vi "VisualizeSiemensDigitalEnergyMeter.vi"() -> ()   [LabVIEW 2018, in "Visualization.lvlib" / "VisualizeSensor.lvclass"]
doc: "This VI listens for any measurement data associated with the provided PluginName and displays it to the user for analysis. The display is only suitable for data coming from the Siemens Plugin."
uses:
  VisualizeSensor.lvclass
  Sensor/SensorShared/clSensorData.ctl
  <extravilib>/ChannelInstances/Tag-bool/Write With Abort.vi
  <extravilib>/ChannelInstances/Tag-bool/Read With Abort.vi
  <extravilib>/ChannelInstances/Tag-bool/Instantiate.vi
  <extravilib>/ChannelInstances/Tag-bool/EndpointRead.vi
  <vilib>/Utility/error.llb/Error Cluster From Error Code.vi
  <extravilib>/ChannelInstances/Tag-bool/Endpoint.vi
  <vilib>/ErrorRing/Error Ring.xnode
  <userlib>/NIST/NISTErrorLib/NISTErrorLib.lvlib
  VisualizeBase/VisualizeBase_class/VisualizeBase.lvclass
  Sensor/SensorShared/SensorShared.lvlib
  Sensor/SensorModule/SensorModule.lvlib
  <extravilib>/ChannelInstances/Tag-bool.lvlib
  TestClass/Test.lvclass
panel:
  in  "ModuleID":i32
  in  "Log Data":bool=TRUE
  in  "btnStop":bool
  in  "btnReset":bool
  in  "btnClearTest":bool
  out "Siemens":waveform(dbl)[](graph)=[{"t0"=timestamp(3657200531.6397257 s since 1904-01-01), "dt"=1.0, "Y"=[46.19]}, {"t0"=timestamp(3657200531.6397257 s since 1904-01-01), "dt"=1.0, "Y"=[2.0]}, {"t0"=timestamp(3657200531.6397257 s since 1904-01-01), "dt"=1.0, "Y"=[60.0]}]
  out "ErrorArray":errorcluster[](array[cluster])
  out "Incorrect DataType?":bool
  out "String Results":string="Sensor.RoomAlert1"
  in  "PluginName":string="Sensor.RoomAlert1"
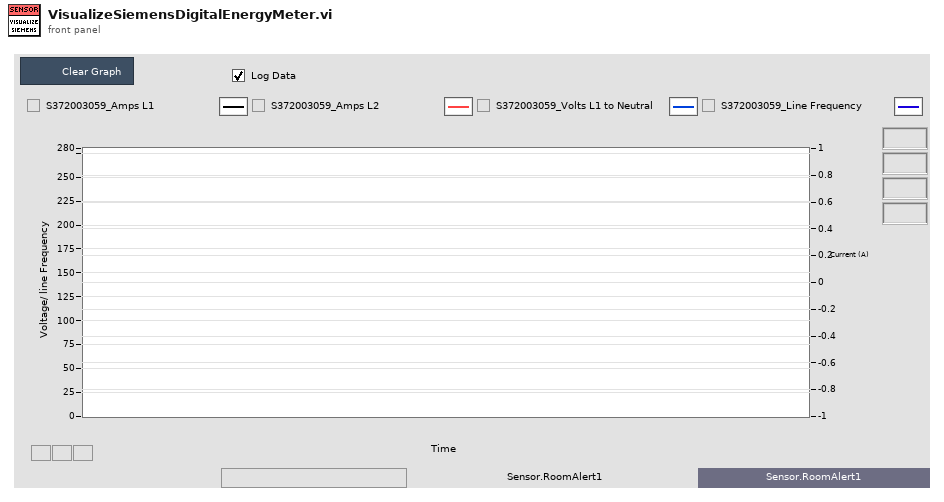
[diagram p1: front panel]
types:
  T1 = enum16{"open", "open or create", "create or replace", "create", "open (read-only)"}
  T2 = typedef "Visualization.lvlib/VisualizeBase.lvclass/clRequestEvents.ctl" = cluster{"StopRequest":refnum<user-event>, "ResetRequest":refnum<user-event>, "FP Pop In or Out":refnum<user-event>}
  T3 = typedef "SensorShared.lvlib/clBroadcastEvents.ctl" = cluster{"DidInit":refnum<user-event>, "StatusUpdate":refnum<user-event>, "ErrorReport":refnum<user-event>, "DidStop":refnum<user-event>, "PathToINI":refnum<user-event>, "SensorReport":refnum<user-event>, "SensorConfig":refnum<user-event>}
  T4 = typedef "SensorShared.lvlib/clSensorData.ctl" = cluster{"SensorType":string, "SensorData":variant}
  T5 = typedef "Tag-bool.lvlib/))Channel.ctl" = refnum<queue>
  T6 = typedef "sizeaction.ctl" = enum32{"Minimized", "Maximized", "Resized"}
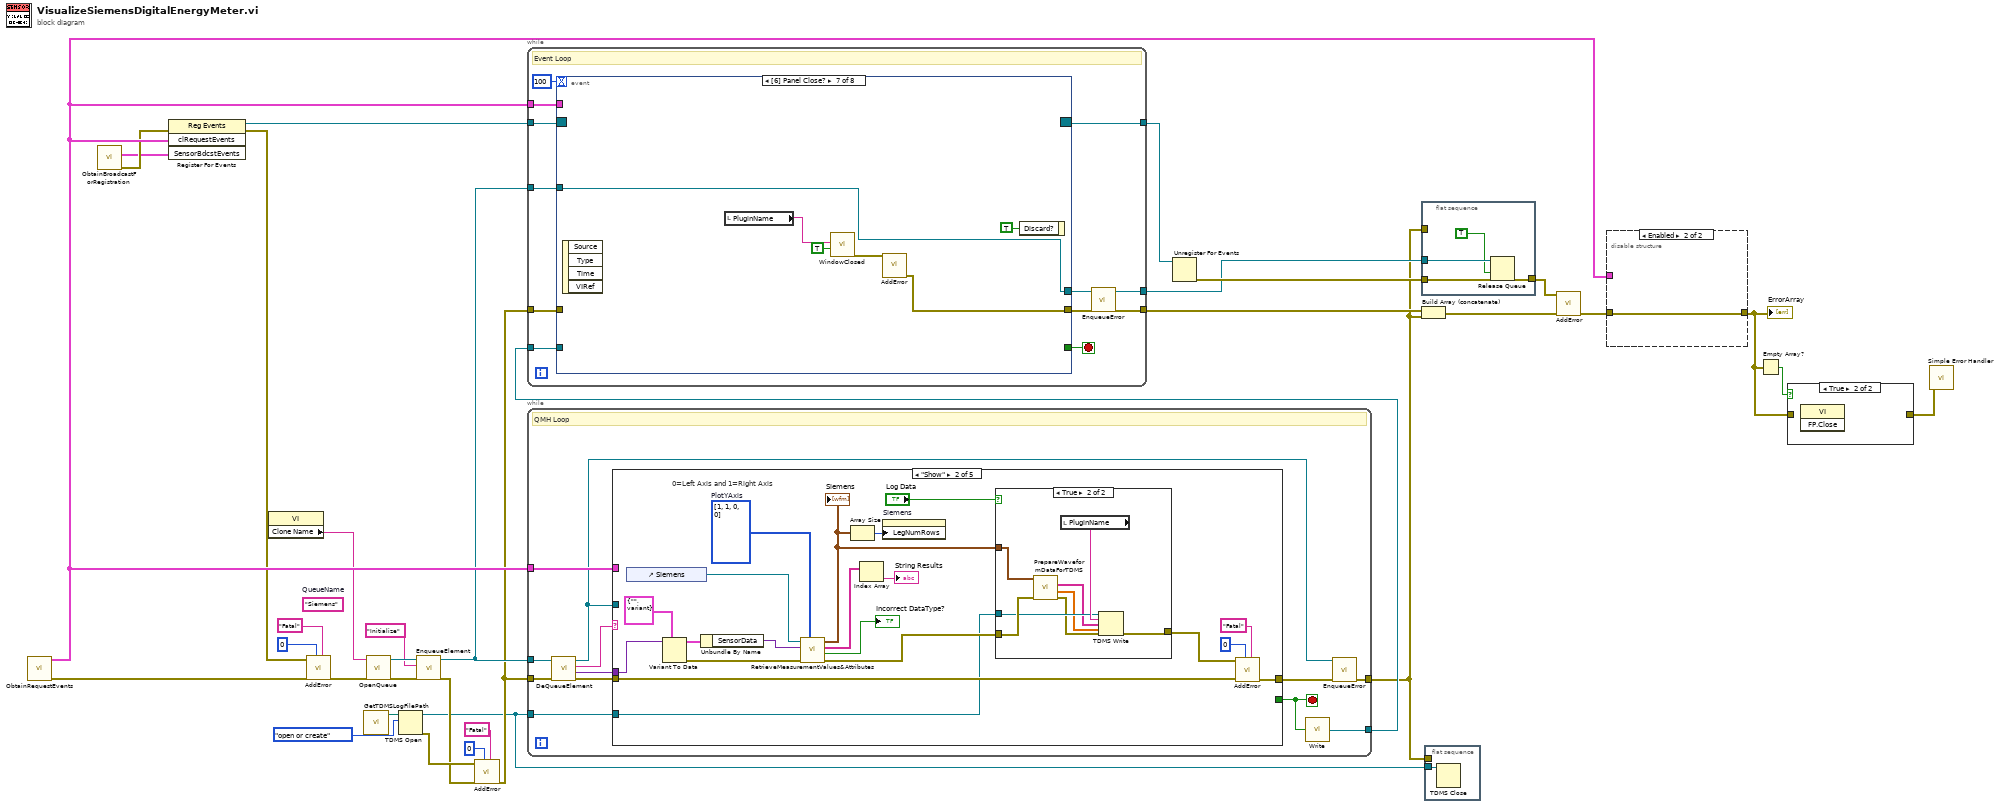
[diagram p0: block diagram]
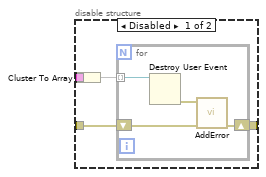
[diagram p2: hidden frame]
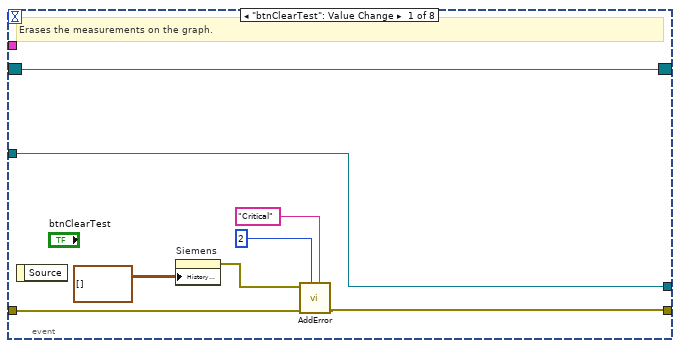
[diagram p3: hidden frame]
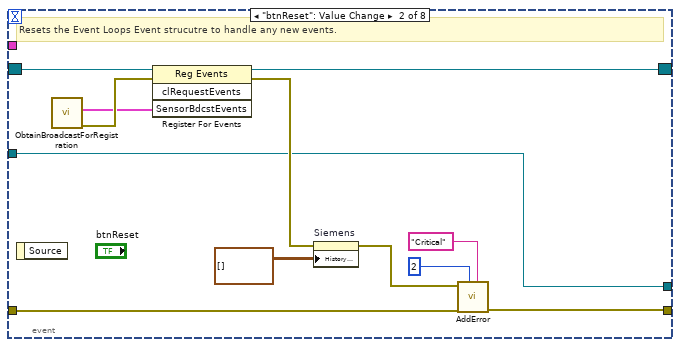
[diagram p4: hidden frame]
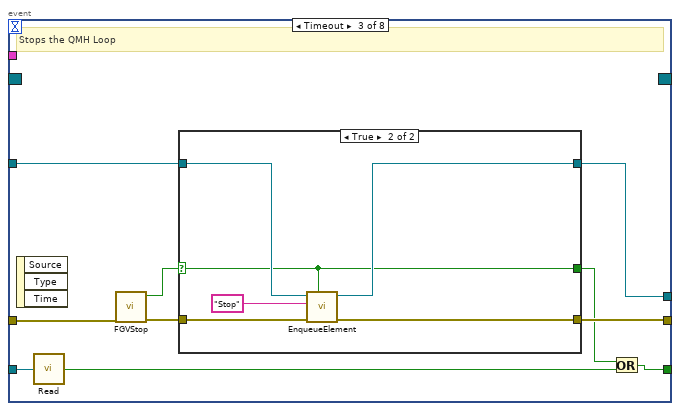
[diagram p5: hidden frame]
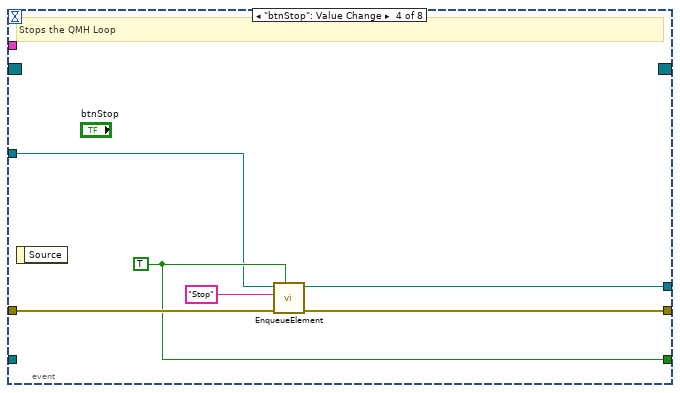
[diagram p7: hidden frame]
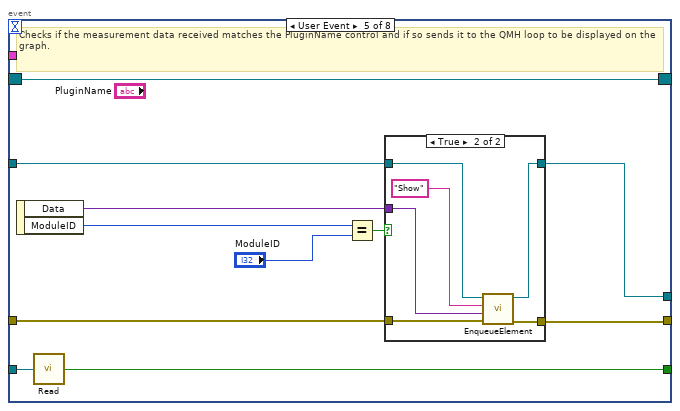
[diagram p8: hidden frame]
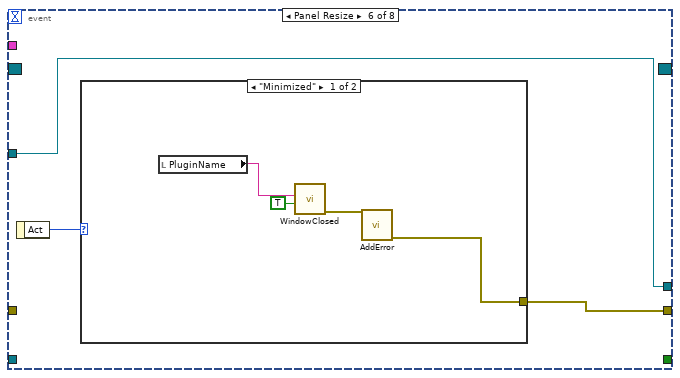
[diagram p10: hidden frame]
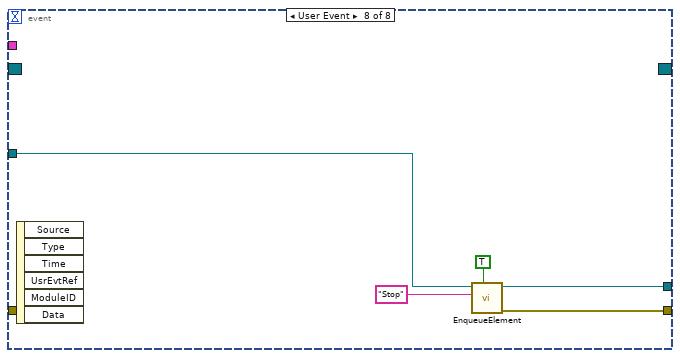
[diagram p12: hidden frame]
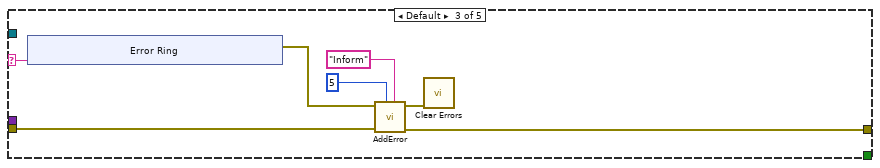
[diagram p15: hidden frame]
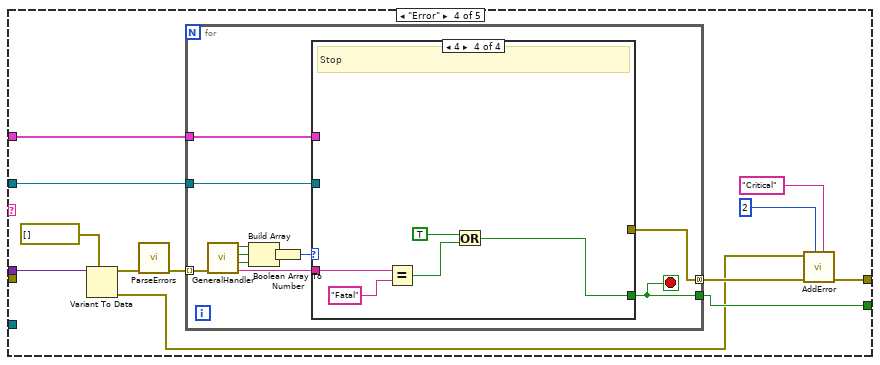
[diagram p16: hidden frame]
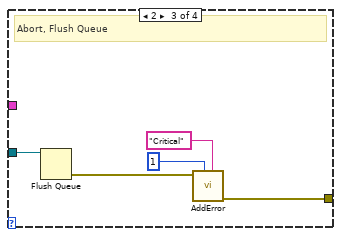
[diagram p19: hidden frame]
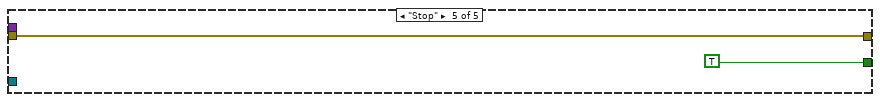
[diagram p20: hidden frame]
diagram:
  (unwired) "Siemens"  # QueueName
  n1 = call "ObtainRequestEvents.vi"() -> ("Error"=w25:errorcluster[], "clRequestEvents"=w27:T2)  [unwired: 10 in]
  n2 = call "ObtainBroadcastForRegistration.vi"() -> ("error out"=w21:errorcluster, "SensorBdcstEvents"=w12:T3)  [unwired: 10 in]
  n3 = register-events(error in=w21, w27, w12) -> (reference out=w34:refnum<event-registration>, error out=w24:errorcluster)  [unwired: 1 in]
  n4 = property class="VI"() -> ("Clone Name"=w10:string)  [unwired: 2 in, 2 out]
  n5 = call <userlib>:"AddError.vi"("Severity"="Fatal", "Priority"=u8 0, "ErrorArray In"=w25, "error in (no error)"=w24) -> ("ErrorArray Out"=w20:errorcluster[])  [unwired: 6 in, 1 out]
  n6 = call "GetTDMSLogFilePath.vi"() -> ("TDMS Log File Path"=w9:path)  [unwired: 11 in]
  n7 = call "OpenQueue.vi"("Error Array In"=w20, "QueueName"=w10) -> ("Error Array Out"=w18:errorcluster[], "queue out"=w19:refnum<queue>)  [unwired: 8 in]
  n8 = TDMS Open(10:T1."open or create" ("operation (0:open)"), 11:w9) -> (0:w5:errorcluster, 3:w2:refnum<k34>)  [unwired: 5 in]
  n9 = call "EnqueueElement.vi"("Error Array In"=w18, "Message"="Initialize", "queue in"=w19) -> ("Error Array Out"=w3:errorcluster[], "queue out"=w16:refnum<queue>)  [unwired: 7 in]
  n10 = call <userlib>:"AddError.vi"("Severity"="Fatal", "Priority"=u8 0, "ErrorArray In"=w3, "error in (no error)"=w5) -> ("ErrorArray Out"=w4:errorcluster[])  [unwired: 6 in, 1 out]
  n11 = while {
    tunnel: w4 -> [w40]
    tunnel: [w43] -> w1
    tunnel: w16 -> [w39]
    tunnel: w27 -> [w45]
    tunnel: [w36] -> w11
    tunnel: w2 -> [w35]
    stop <- w46 stop-if-true
    # "QMH Loop"
    n12 = call "DeQueueElement.vi"("Error Array In"=w40, "Queue In"=w39) -> ("Error Array Out"=w38:errorcluster[], "Data"=w41:variant, "Message"=w42:string, "Queue Out"=w37:refnum<queue>)  [unwired: 6 in]
    n13 = case shown="\"Show\"" w42 {
      selector: w42 -> [_ _ w83 _ _]
      tunnel: w41 -> [_ w61 _ w102 _]
      tunnel: w38 -> [w47 w65 w81 _ w124]
      tunnel: [w47 w67 w80 w92 w124] -> w44
      tunnel: [_ _ _ w98 TRUE] -> w46
      tunnel: w45 -> [_ _ _ w97 _]
      tunnel: w37 -> [_ _ _ w96 _]
      tunnel: w35 -> [_ w50 _ _ _]
      frame "Initialize" {
      }
      frame "Show" {
        w58 = u32[] [1, 1, 0, 0]  # PlotYAxis
        # "0=Left Axis and 1=Right Axis"
        n14 = control-ref of="Siemens"() -> (w66:refnum<vi>)
        n15 = Variant To Data(type=T4 {"SensorType"="", "SensorData"=variant} ("clSensorData"), Variant=w61) -> (data=w59:T4, error out=w60:errorcluster)  [unwired: 1 in]
        n16 = Unbundle By Name(w59) -> ("SensorData"=w56:variant)
        n17 = call "RetrieveMeasurementValues&Attributes.vi"("PlotYScale"=w58, "error in (no error)"=w60, "Variant"=w56, "WaveformChartReference"=w66) -> ("error out"=w55:errorcluster, "Incorrect DataType?"=→"Incorrect DataType?":bool, "Array Of Strings"=w52:string[], "WaveformArrayOut"=w48:waveform(dbl)[])  [unwired: 3 in, 1 out]
        "Siemens" <- w48
        n18 = Array Size(array=w48) -> (size(s)=w49:i32)
        n19 = Index Array(array=w52) -> (element=→"String Results":string)  [unwired: 1 in]
        n20 = property on="Siemens" class="WFChart (strict)"("LegNumRows"=w49) -> ()  [unwired: 2 in, 2 out]
        n21 = case shown="True" "Log Data" {
          tunnel: w55 -> [w68 w76]
          tunnel: [w68 w74] -> w54
          tunnel: w48 -> [_ w71]
          tunnel: w50 -> [_ w73]
          frame False {
          }
          frame True {
            n22 = call "PrepareWaveformDataForTDMS.vi"("error in (no error)"=w76, "WaveformArray in"=w71) -> ("error out"=w72:errorcluster, "Measurement Data"=w69:dbl[][], "Channel Names"=w70:string[])  [unwired: 7 in]
            n23 = local read "PluginName"() -> (w75:string)
            n24 = TDMS Write(0:w73, 5:w75, 7:w70, 9:w69, 11:w72) -> (15:w74:errorcluster)  [unwired: 1 in, 3 out]
          }
        }
        n25 = call <userlib>:"AddError.vi"("Severity"="Fatal" ("String"), "Priority"=u8 0, "ErrorArray In"=w65, "error in (no error)"=w54) -> ("ErrorArray Out"=w67:errorcluster[])  [unwired: 6 in, 1 out]
      }
      frame Default {
        n26 = xnode "Error Ring"("parameter 0"=w83) -> ("error out"=w82:errorcluster)
        n27 = call <userlib>:"AddError.vi"("Severity"="Inform" ("String"), "Priority"=u8 5, "ErrorArray In"=w81, "error in (no error)"=w82) -> ("ErrorArray Out"=w80:errorcluster[], "error out"=w79:errorcluster)  [unwired: 6 in]
        n28 = call <vilib>:"Clear Errors.vi"("error in (no error)"=w79) -> ()  [unwired: 5 in, 2 out]
      }
      frame "Error" {
        n29 = Variant To Data(type=errorcluster[] [], Variant=w102) -> (data=w100:errorcluster[], error out=w91:errorcluster)  [unwired: 1 in]
        n30 = call <userlib>:"ParseErrors.vi"("ErrorArray"=w100) -> ("ErrorArray"=w99:errorcluster[])  [unwired: 8 in, 2 out]
        n31 = for {
          tunnel: w99 -> [w113] mode=indexing
          tunnel: [w107] -> w93 mode=concatenating
          tunnel: [w105] -> w98
          tunnel: w97 -> [w104]
          tunnel: w96 -> [w103]
          stop <- w105 stop-if-true
          n32 = call <userlib>:"GeneralHandler.vi"("error in (no error)"=w113) -> ("Severity"=w106:string, "Stop"=w110:bool, "Abort"=w111:bool, "Continue"=w112:bool)  [unwired: 6 in, 1 out]
          n33 = Build Array(w112, w111, w110) -> (w109:bool[])
          n34 = Boolean Array To Number(Boolean array=w109) -> (number=w108:u32)
          n35 = case shown="4" w108 {
            tunnel: [_ _ w118 _] -> w107
            tunnel: w106 -> [_ _ _ w123]
            tunnel: [_ _ _ w119] -> w105
            tunnel: w104 -> [_ _ _ _]
            tunnel: w103 -> [_ _ w114 _]
            frame 0, Default {
              # "No Dialog"
            }
            frame 1 {
              # "Continue"
            }
            frame 2 {
              # "Abort, Flush Queue"
              n36 = Flush Queue(queue=w114) -> (error out=w117:errorcluster)  [unwired: 1 in, 2 out]
              n37 = call <userlib>:"AddError.vi"("Severity"="Critical" ("String"), "Priority"=u8 1, "error in (no error)"=w117) -> ("ErrorArray Out"=w118:errorcluster[])  [unwired: 7 in, 1 out]
            }
            frame 4 {
              # "Stop"
              n38 = Equal?(x=w123, y="Fatal" ("x")) -> (x = y?=w120:bool)
              n39 = Or(x=TRUE, y=w120) -> (x .or. y?=w119:bool)
            }
          }
        }
        n40 = call <userlib>:"AddError.vi"("Severity"="Critical", "Priority"=u8 2, "ErrorArray In"=w93, "error in (no error)"=w91) -> ("ErrorArray Out"=w92:errorcluster[])  [unwired: 6 in, 1 out]
      }
      frame "Stop" {
      }
    }
    n41 = call <extravilib>:"Write.vi"("element"=w46) -> ("channel"=w36:T5)  [unwired: 1 out]
    n42 = call "EnqueueError.vi"("Error Array In"=w44, "Queue in"=w37) -> ("Error Array Out"=w43:errorcluster[])  [unwired: 8 in, 1 out]
  }
  n43 = while {
    tunnel: w34 -> [w137]
    tunnel: [w131] -> w32
    tunnel: [w135] -> w33
    tunnel: w27 -> [w134]
    tunnel: w4 -> [w133]
    tunnel: w16 -> [w132]
    tunnel: [w128] -> w15
    tunnel: w11 -> [w126]
    stop <- w136 stop-if-true
    # "Event Loop"
    n44 = event shown="[6] Panel Close?" {
      selector: w137 -> [w139 w157 _ _ w189 _ _ _]
      dyn-events: [w139 w156 _ _ w189 _ _ _] -> w135
      timeout: 100 -> [_ _ _ _ _ _ _ _]
      tunnel: [_ _ w161 w179 w185 _ _ _] -> w136
      tunnel: [w142 w154 w163 w181 w191 w203 w210 w215] -> w130
      tunnel: w134 -> [_ _ _ _ _ _ _ _]
      tunnel: w133 -> [w143 w155 w164 w182 w192 _ _ _]
      tunnel: w132 -> [w138 w147 w160 w177 w193 w202 w209 w217]
      tunnel: [w138 w147 w159 w180 w190 w202 w209 w216] -> w129
      tunnel: w126 -> [_ _ w167 _ w186 _ _ _]
      event "btnClearTest": Value Change {
        # "Erases the measurements on the graph."
        n45 = event-data() -> ()  [unwired: 1 in, 1 out]
        n46 = property on="Siemens" class="WFChart (strict)"("History Data"=waveform(dbl)[][] []) -> (error out=w141:errorcluster)  [unwired: 2 in, 1 out]
        n47 = call <userlib>:"AddError.vi"("Severity"="Critical", "Priority"=u8 2, "ErrorArray In"=w143, "error in (no error)"=w141) -> ("ErrorArray Out"=w142:errorcluster[])  [unwired: 6 in, 1 out]
      }
      event "btnReset": Value Change {
        # "Resets the Event Loops Event strucutre to handle any new events."
        n48 = event-data() -> ()  [unwired: 1 in, 1 out]
        n49 = call "ObtainBroadcastForRegistration.vi"() -> ("error out"=w148:errorcluster, "SensorBdcstEvents"=w146:T3)  [unwired: 10 in]
        n50 = register-events(reference=w157, error in=w148, w146) -> (reference out=w156:refnum<event-registration>, error out=w150:errorcluster)  [unwired: 1 in]
        n51 = property on="Siemens" class="WFChart (strict)"(error in=w150, "History Data"=waveform(dbl)[][] []) -> (error out=w149:errorcluster)  [unwired: 1 in, 1 out]
        n52 = call <userlib>:"AddError.vi"("Severity"="Critical", "Priority"=u8 2, "ErrorArray In"=w155, "error in (no error)"=w149) -> ("ErrorArray Out"=w154:errorcluster[])  [unwired: 6 in, 1 out]
      }
      event Timeout {
        # "Stops the QMH Loop"
        n53 = event-data() -> ()  [unwired: 1 in, 3 out]
        n54 = call <extravilib>:"Read.vi"("channel"=w167) -> ("element"=w162:bool)  [unwired: 1 in, 1 out]
        n55 = call "FGVStop.vi"("Error In"=w164) -> ("Error Out"=w165:errorcluster[], "Value"=w166:bool)  [unwired: 9 in]
        n56 = case shown="True" w166 {
          selector: w166 -> [w168 w171]
          tunnel: [w170 w174] -> w163
          tunnel: w165 -> [w170 w175]
          tunnel: w160 -> [w169 w173]
          tunnel: [w169 w172] -> w159
          tunnel: [w168 w171] -> w158
          frame False {
          }
          frame True {
            n57 = call "EnqueueElement.vi"("Priority? (F)"=w171, "Error Array In"=w175, "Message"="Stop", "queue in"=w173) -> ("Error Array Out"=w174:errorcluster[], "queue out"=w172:refnum<queue>)  [unwired: 6 in]
          }
        }
        n58 = Or(x=w158, y=w162) -> (x .or. y?=w161:bool)
      }
      event "btnStop": Value Change {
        w179 = TRUE ("Priority? (F)")
        # "Stops the QMH Loop"
        n59 = event-data() -> ()  [unwired: 1 in, 1 out]
        n60 = call "EnqueueElement.vi"("Priority? (F)"=w179, "Error Array In"=w182, "Message"="Stop", "queue in"=w177) -> ("Error Array Out"=w181:errorcluster[], "queue out"=w180:refnum<queue>)  [unwired: 6 in]
      }
      event User Event {
        # "Checks if the measurement data received matches the PluginName control and if so sends it to the QMH loop to be displayed on the graph."
        n61 = event-data() -> ("Data"=w188:variant, "ModuleID"=w183:i32)  [unwired: 1 in]
        n62 = call <extravilib>:"Read.vi"("channel"=w186) -> ("element"=w185:bool)  [unwired: 1 in, 1 out]
        n63 = Equal?(x=w183, y="ModuleID") -> (x = y?=w187:bool)
        n64 = case shown="True" w187 {
          tunnel: [w194 w200] -> w191
          tunnel: w193 -> [w195 w199]
          tunnel: w192 -> [w194 w201]
          tunnel: [w195 w197] -> w190
          tunnel: w188 -> [_ w198]
          frame False {
          }
          frame True {
            n65 = call "EnqueueElement.vi"("Error Array In"=w201, "Data"=w198, "Message"="Show", "queue in"=w199) -> ("Error Array Out"=w200:errorcluster[], "queue out"=w197:refnum<queue>)  [unwired: 6 in]
          }
        }
      }
      event Panel Resize {
        n66 = event-data() -> ("Act"=w204:T6)  [unwired: 1 in]
        n67 = case shown="\"Minimized\"" w204 {
          tunnel: [w205 _] -> w203
          frame "Minimized" {
            n68 = local read "PluginName"() -> (w207:string)
            n69 = call "WindowClosed.vi"("Window Closed?"=TRUE ("Window Minimized or Clozed?"), "Module Name"=w207) -> ("error out"=w208:errorcluster)  [unwired: 9 in]
            n70 = call <userlib>:"AddError.vi"("error in (no error)"=w208) -> ("ErrorArray Out"=w205:errorcluster[])  [unwired: 9 in, 1 out]
          }
          frame "Maximized", Default {
          }
        }
      }
      event Panel Close? {
        n71 = event-data() -> ()  [unwired: 1 in, 4 out]
        n72 = local read "PluginName"() -> (w211:string)
        n73 = call "WindowClosed.vi"("Window Closed?"=TRUE ("Window Minimized or Clozed?"), "Module Name"=w211) -> ("error out"=w213:errorcluster)  [unwired: 9 in]
        n74 = call <userlib>:"AddError.vi"("error in (no error)"=w213) -> ("ErrorArray Out"=w210:errorcluster[])  [unwired: 9 in, 1 out]
        n75 = event-data("Discard?"=TRUE) -> ()  [unwired: 1 in, 1 out]
      }
      event User Event {
        n76 = event-data() -> ()  [unwired: 1 in, 6 out]
        n77 = call "EnqueueElement.vi"("Priority? (F)"=TRUE, "Message"="Stop", "queue in"=w217) -> ("Error Array Out"=w215:errorcluster[], "queue out"=w216:refnum<queue>)  [unwired: 7 in]
      }
    }
    n78 = call "EnqueueError.vi"("Error Array In"=w130, "Queue in"=w129) -> ("Error Array Out"=w131:errorcluster[], "Queue out"=w128:refnum<queue>)  [unwired: 8 in]
  }
  n79 = Unregister For Events(event registration refnum=w33) -> (error out=w31:errorcluster)  [unwired: 1 in]
  n80 = flat-sequence {
    tunnel: w31 -> [w223]
    tunnel: [w222] -> w29
    tunnel: w15 -> [w221]
    tunnel: w1 -> [_]
    frame #0 {
      n81 = Release Queue(queue=w221, force destroy? (F)=TRUE, error in (no error)=w223) -> (error out=w222:errorcluster)  [unwired: 2 out]
    }
  }
  n82 = Build Array (concatenate)(w32, w1) -> (w30:errorcluster[])
  n83 = flat-sequence {
    tunnel: w2 -> [w224]
    tunnel: w1 -> [_]
    frame #0 {
      n84 = TDMS Close(11:w224) -> ()  [unwired: 1 in, 2 out]
    }
  }
  n85 = call <userlib>:"AddError.vi"("ErrorArray In"=w30, "error in (no error)"=w29) -> ("ErrorArray Out"=w28:errorcluster[])  [unwired: 8 in, 1 out]
  n86 = disable-structure shown="Enabled" {
    disable-tunnel: w28 -> [w227 w233]
    disable-tunnel: w27 -> [w226 _]
    disable-tunnel: [w225 w233] -> w14
    frame Disabled {
      n87 = Cluster To Array(cluster=w226) -> (array=w228:refnum<user-event>[])
      n88 = for {
        tunnel: w228 -> [w232] mode=indexing
        shift-right: [w231] -> w225
        shift-left: w227 -> [w230]
        n89 = Destroy User Event(user event=w232) -> (error out=w229:errorcluster)  [unwired: 1 in]
        n90 = call <userlib>:"AddError.vi"("ErrorArray In"=w230, "error in (no error)"=w229) -> ("ErrorArray Out"=w231:errorcluster[])  [unwired: 8 in, 1 out]
      }
    }
    frame Enabled {
    }
  }
  "ErrorArray" <- w14
  n91 = Empty Array?(array=w14) -> (empty?=w26:bool)
  n92 = case shown="True" w26 {
    tunnel: [w234 _] -> w13
    tunnel: w14 -> [w235 _]
    frame False {
      n93 = Merge Errors(w235) -> (w234:errorcluster)
    }
    frame True {
      n94 = invoke class="VI" method="FP.Close"() -> ()  [unwired: 3 in, 3 out]
    }
  }
  n95 = call <vilib>:"Simple Error Handler.vi"("error in (no error)"=w13) -> ()  [unwired: 4 in, 5 out]
